vi "Initialize.vi"(7 "Serial Configuration":T1={"Baud Rate"=115200, "Parity"=0, "Data Bits"=8, "Stop Bits"=10, "Flow Control"=0} {"Flow Control" items=["None", "XON/XOFF", "RTS/CTS", "XON/XOFF & RTS/CTS", "DTR/DSR", "XON/XOFF & DTR/DSR"]; "Stop Bits" items=["1.0"=10, "1.5"=15, "2.0"=20]; "Data Bits" items=["7"=7, "8"=8]; "Parity" items=["None", "Odd", "Even", "Mark", "Space"]; "Baud Rate" items=["300"=300, "600"=600, "1200"=1200, "2400"=2400, "4800"=4800, "9600"=9600, "19200"=19200, "115200"=115200]}, 8 "error in (no error)":errorcluster, 9 "Reset (True)":bool=TRUE, 10 "ID Query (True)":bool=TRUE, 11 "VISA resource name":refnum<visa-resource-name>) -> (0 "error out":errorcluster, 3 "VISA resource name out":refnum<visa-resource-name>)   [LabVIEW 2013, in "HadCon.lvlib"]
doc: "Establishes communication with the instrument and optionally performs an instrument identification query and/or an instrument reset. It also places the instrument in a default state needed for other instrument driver operations. Therefore, call this VI before calling other instrument driver VIs for this instrument. Generally, you need to call the Initialize VI only once at the beginning of an application."
uses:
  <instrlib>/HadCon/HadCon.lvlib
panel:
  # "(c) 2014 GSI Helmholtzzentrum für Schwerionenforschung GmbH.  ALL RIGHTS RESERVED."
  # "Licensed under EUPL V. 1.1"
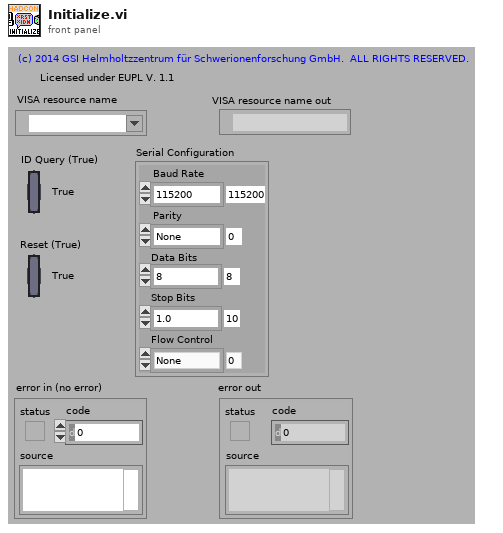
[diagram p1: front panel]
types:
  T1 = cluster{"Baud Rate":u32, "Parity":u16, "Data Bits":u16, "Stop Bits":u16, "Flow Control":u16}
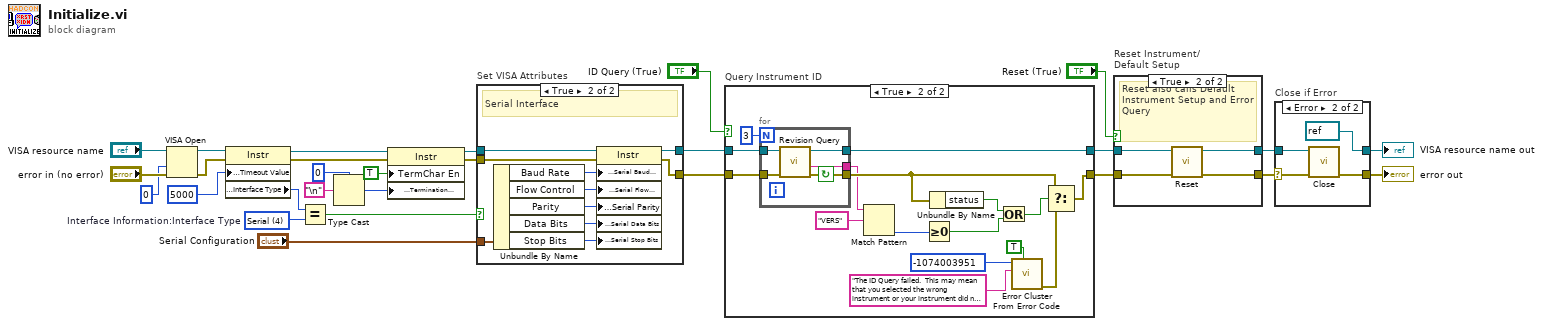
[diagram p0: block diagram]
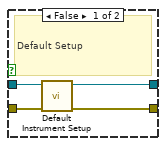
[diagram p4: hidden frame]
diagram:
  w15 = u16 4 items=["GPIB"=1, "VXI"=2, "GPIB-VXI"=3, "Serial"=4, "PXI"=5, "TCPIP"=6, "USB"=7]  # Interface Information:Interface Type
  n1 = VISA Open(access mode=u32 0, error in (no error)="error in (no error)", VISA resource name="VISA resource name") -> (VISA resource name=w9:refnum<visa-resource-name>, error out=w8:errorcluster)  [unwired: 2 in]
  n2 = property class="Instr"(reference=w9, error in=w8, "General Settings:Timeout Value"=u32 5000) -> (reference out=w1:refnum<visa-resource-name>, error out=w17:errorcluster, "Interface Information:Interface Type"=w21:u16)
  n3 = Equal?(x=w21, y=w15) -> (x = y?=w16:bool)
  n4 = Type Cast(type=u8 0, x="\n") -> (*(type *) &x=w5:u8)
  n5 = property class="Instr"(reference=w1, "TermChar En"=TRUE ("Message Based Settings:Termination Character Enable"), "Message Based Settings:Termination Character"=w5) -> (reference out=w2:refnum<visa-resource-name>)  [unwired: 1 in, 1 out]
  n6 = case "Set VISA Attributes" shown="True" w16 {
    tunnel: [w28 w32] -> w19
    tunnel: [w29 w31] -> w18
    tunnel: w2 -> [w28 w38]
    tunnel: w17 -> [w29 w39]
    tunnel: "Serial Configuration" -> [_ w30]
    frame False {
      # "TCP/IP"
    }
    frame True {
      # "Serial Interface"
      n7 = Unbundle By Name(w30) -> ("Baud Rate"=w37:u32, "Flow Control"=w34:u16, "Parity"=w35:u16, "Data Bits"=w36:u16, "Stop Bits"=w33:u16)
      n8 = property class="Instr"(reference=w38, error in=w39, "Serial Settings:Serial Baud Rate"=w37, "Serial Settings:Serial Flow Control"=w34, "Serial Settings:Serial Parity"=w35, "Serial Settings:Serial Data Bits"=w36, "Serial Settings:Serial Stop Bits"=w33) -> (reference out=w32:refnum<visa-resource-name>, error out=w31:errorcluster)
    }
  }
  n9 = case "Query Instrument ID" shown="True" "ID Query (True)" {
    tunnel: [w40 w57] -> w26
    tunnel: [w41 w45] -> w27
    tunnel: w19 -> [w41 w47]
    tunnel: w18 -> [w40 w46]
    frame False {
    }
    frame True {
      n10 = for {
        N: 3 -> [_]
        tunnel: w47 -> [w62]
        tunnel: w46 -> [w61]
        tunnel: [w60] -> w45
        tunnel: [w58] -> w44
        tunnel: [w59] -> w43
        stop <- w58 continue-if-true
        n11 = call <instrlib>:"Revision Query.vi"("error in (no error)"=w61, "VISA resource name"=w62) -> ("error out"=w58:errorcluster, "Instrument Firmware Revision"=w59:string, "VISA resource name out"=w60:refnum<visa-resource-name>)  [unwired: 6 in, 1 out]
      }
      n12 = Match Pattern(string=w43, regular expression="VERS") -> (offset past match=w51:i32)  [unwired: 1 in, 3 out]
      n13 = Greater Or Equal To 0?(x=w51) -> (x >= 0?=w49:bool)
      n14 = Unbundle By Name(w44) -> ("status"=w50:bool)
      n15 = Or(x=w50, y=w49) -> (x .or. y?=w48:bool)
      n16 = call <vilib>:"Error Cluster From Error Code.vi"("show call chain? (False)"=TRUE, "error message (\"\")"="The ID Query failed.  This may mean that you selected the wrong instrument or your instrument did not respond.  You may also be using a model that is not officially supported by this driver.  If you are sure that you have selected the correct instrument and it is responding, try disabling the ID Query." ("Source (VI Name)"), "error code (0)"=-1074003951 ("Code")) -> ("error out"=w55:errorcluster)  [unwired: 6 in]
      n17 = Select(t=w44, s=w48, f=w55) -> (s? t:f=w57:errorcluster)
    }
  }
  n18 = case "Reset Instrument/\nDefault Setup" shown="True" "Reset (True)" {
    tunnel: w26 -> [w65 w67]
    tunnel: [w63 w70] -> w10
    tunnel: w27 -> [w66 w68]
    tunnel: [w64 w69] -> w11
    frame False {
      # "Default Setup"
      n19 = call <instrlib>:"Default Instrument Setup.vi"("error in (no error)"=w65, "VISA resource name"=w66) -> ("error out"=w63:errorcluster, "VISA resource name out"=w64:refnum<visa-resource-name>)  [unwired: 8 in]
    }
    frame True {
      # "Reset also calls Default Instrument Setup and Error Query"
      n20 = call <instrlib>:"Reset.vi"("error in (no error)"=w67, "VISA resource name"=w68) -> ("error out"=w70:errorcluster, "VISA resource name out"=w69:refnum<visa-resource-name>)  [unwired: 8 in]
    }
  }
  n21 = case "Close if Error" shown="Error" w10 {
    selector: w10 -> [w71 w74]
    tunnel: w11 -> [w72 w75]
    tunnel: [w72 refnum<visa-resource-name> refnum ("VISA resource name out")] -> w13
    tunnel: [w71 w76] -> w12
    frame No Error {
    }
    frame Error {
      n22 = call <instrlib>:"Close.vi"("error in (no error)"=w74, "VISA resource name"=w75) -> ("error out"=w76:errorcluster)  [unwired: 9 in]
    }
  }
  "VISA resource name out" <- w13
  "error out" <- w12
